vi "WriteSetPointCode SubVI.vi"(1 "SetPointCode 2":u16) -> (0 "SetPointCode":u8)   [LabVIEW 2019]
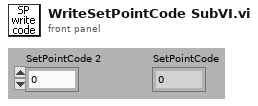
[diagram p1: front panel]
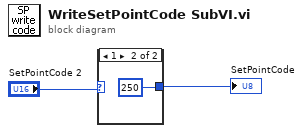
[diagram p0: block diagram]
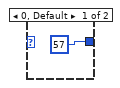
[diagram p2: hidden frame]
diagram:
  n1 = case shown="1" "SetPointCode 2" {
    tunnel: [u8 57 u8 250] -> w2
    frame 0, Default {
    }
    frame 1 {
    }
  }
  "SetPointCode" <- w2
